vi "Handle.vi"(8 "error in (no error)":errorcluster, 11 "Instrument in":refnum<class "Instrument.lvclass">) -> (0 "error out":errorcluster, 3 "Instrument out":refnum<class "Instrument.lvclass">)   [LabVIEW 2018, in "Instrument.lvclass"]
uses:
  Instrument.lvclass
  Instrument.lvclass/Instrument.ctl
  Server/Server.lvclass
  Comm/Stream/Stream.lvclass
  Device/Optics/Opt_Selector/Opt_Selector.lvclass
  Device/Optics/Opt_Continuous/Opt_Continuous.lvclass
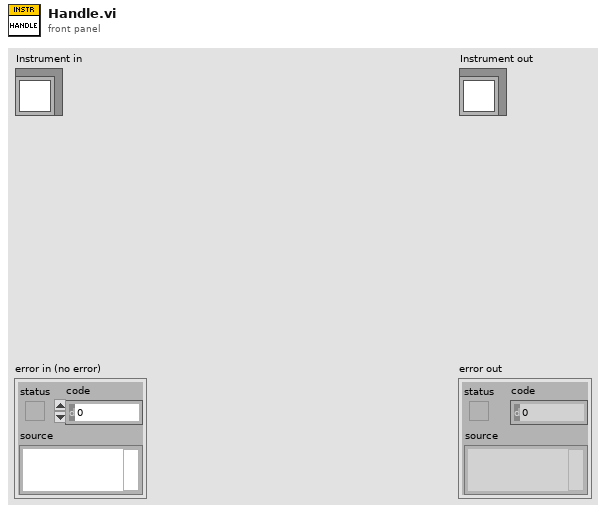
[diagram p1: front panel]
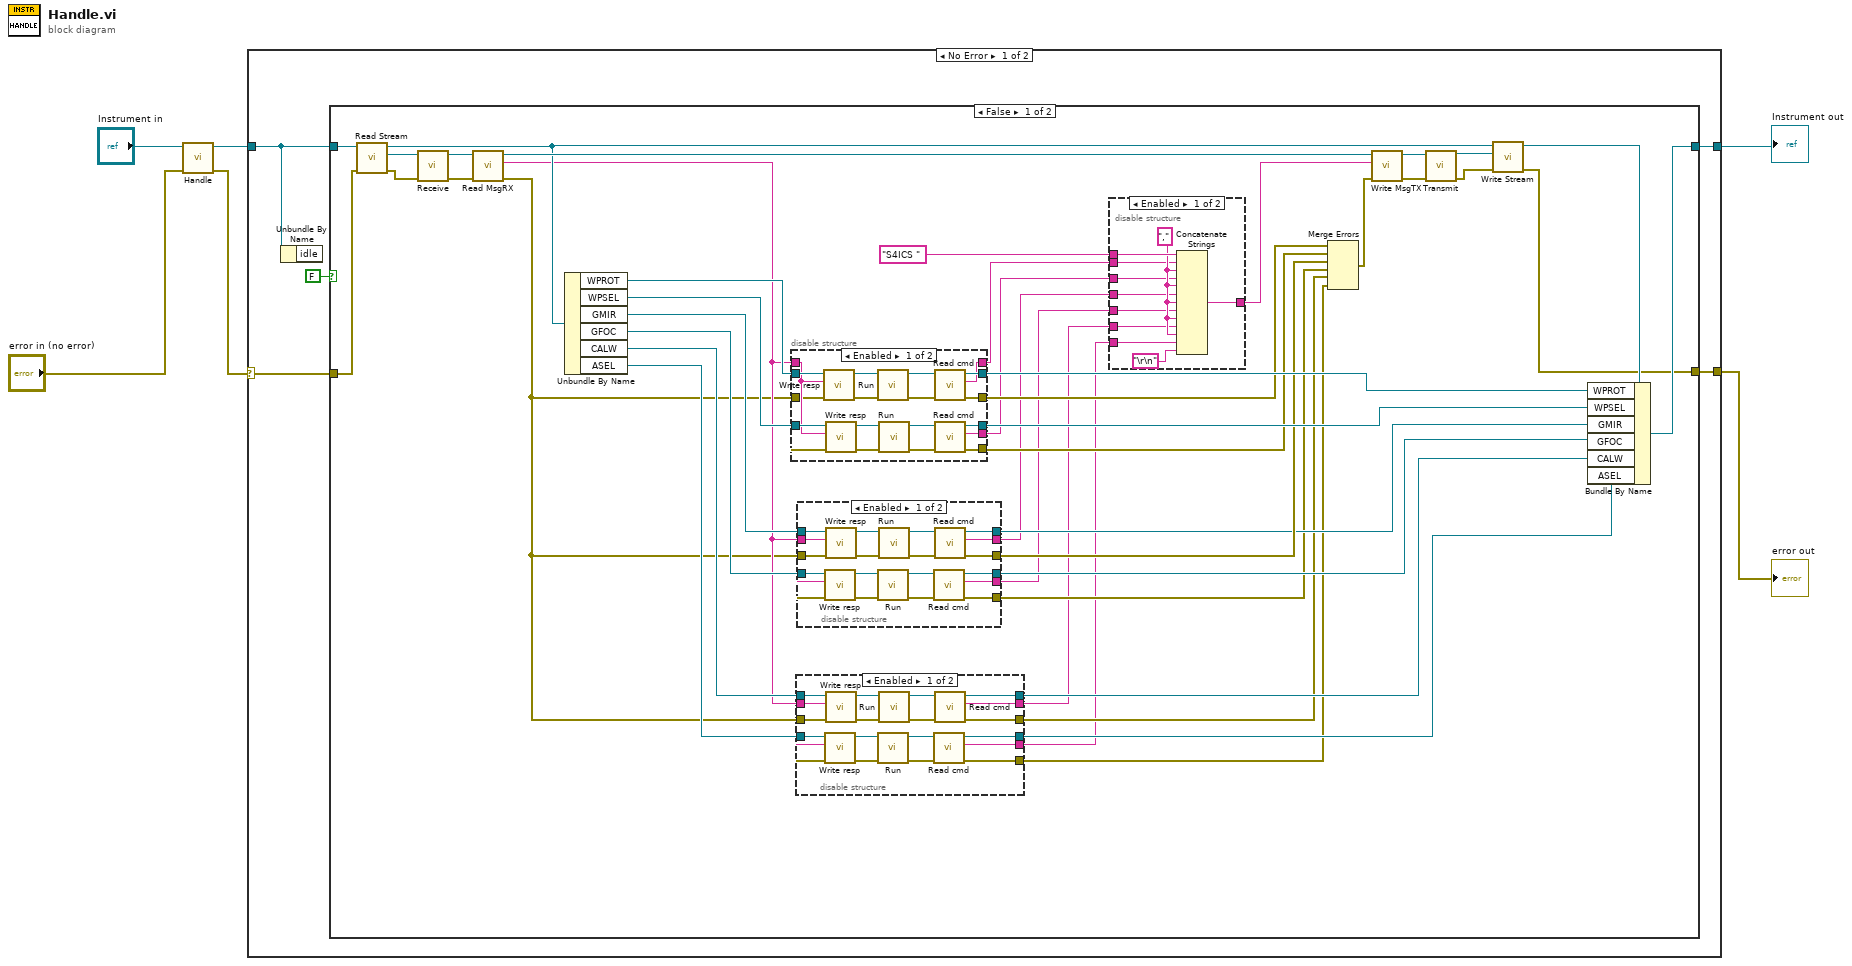
[diagram p0: block diagram]
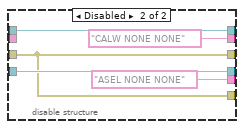
[diagram p2: hidden frame]
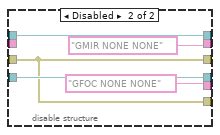
[diagram p3: hidden frame]
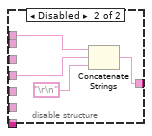
[diagram p4: hidden frame]
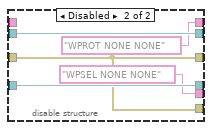
[diagram p5: hidden frame]
diagram:
  n1 = call-parent "Handle.vi"("error in (no error)"="error in (no error)", "Server in"="Instrument in") -> ("error out"=w3:errorcluster, "Server out"=w4:refnum<class "Instrument.lvclass">)  [unwired: 8 in]
  n2 = case shown="No Error" w3 {
    selector: w3 -> [w11 w142]
    tunnel: [w9 w142] -> w2
    tunnel: [w10 w141] -> w1
    tunnel: w4 -> [w8 w141]
    frame No Error {
      n3 = Unbundle By Name(w8) -> ()  [unwired: 1 out]
      n4 = case shown="False" FALSE {
        tunnel: w11 -> [w53 w139]
        tunnel: [w51 w140] -> w10
        tunnel: [w41 w139] -> w9
        tunnel: w8 -> [w19 w140]
        frame False {
          n5 = call-dynamic "Read Stream.vi"("error in (no error)"=w53, "Server in"=w19) -> ("error out"=w54:errorcluster, "Stream.lvclass"=w55:refnum<class "Stream.lvclass">, "Server out"=w45:refnum<class "Instrument.lvclass">)  [unwired: 7 in]
          n6 = call-dynamic "Receive.vi"("error in (no error)"=w54, "Stream in"=w55) -> ("error out"=w50:errorcluster, "Stream out"=w49:refnum<class "Stream.lvclass">)  [unwired: 8 in]
          n7 = call-dynamic "Read MsgRX.vi"("error in (no error)"=w50, "Comm in"=w49) -> ("error out"=w26:errorcluster, "MsgRX"=w27:string, "Comm out"=w48:refnum<class "Stream.lvclass">)  [unwired: 7 in]
          n8 = Unbundle By Name(w45) -> ("WPROT"=w52:refnum<class "Opt_Selector.lvclass">, "WPSEL"=w40:refnum<class "Opt_Selector.lvclass">, "GMIR"=w33:refnum<class "Opt_Continuous.lvclass">, "GFOC"=w30:refnum<class "Opt_Continuous.lvclass">, "CALW"=w29:refnum<class "Opt_Selector.lvclass">, "ASEL"=w28:refnum<class "Opt_Selector.lvclass">)
          n9 = disable-structure shown="Enabled" {
            disable-tunnel: w52 -> [w133 w138]
            disable-tunnel: w40 -> [w128 w137]
            disable-tunnel: [w127 w138] -> w37
            disable-tunnel: [w126 w136] -> w36
            disable-tunnel: [w125 w137] -> w35
            disable-tunnel: [w124 w136] -> w34
            disable-tunnel: w27 -> [w123 _]
            disable-tunnel: w26 -> [w122 w136]
            disable-tunnel: [w121 "WPROT NONE NONE" ("cmd")] -> w18
            disable-tunnel: [w120 "WPSEL NONE NONE" ("cmd")] -> w17
            frame Enabled {
              n10 = call-dynamic "Write resp.vi"("error in (no error)"=w122, "resp"=w123, "Device in"=w133) -> ("error out"=w131:errorcluster, "Device out"=w132:refnum<class "Opt_Selector.lvclass">)  [unwired: 7 in]
              n11 = call-dynamic "Write resp.vi"("error in (no error)"=w122, "resp"=w123, "Device in"=w128) -> ("error out"=w118:errorcluster, "Device out"=w119:refnum<class "Opt_Selector.lvclass">)  [unwired: 7 in]
              n12 = call-dynamic "Run.vi"("error in (no error)"=w131, "Opctics in"=w132) -> ("error out"=w130:errorcluster, "Opt_Selector out"=w129:refnum<class "Opt_Selector.lvclass">)  [unwired: 8 in]
              n13 = call-dynamic "Run.vi"("error in (no error)"=w118, "Opctics in"=w119) -> ("error out"=w117:errorcluster, "Opt_Selector out"=w116:refnum<class "Opt_Selector.lvclass">)  [unwired: 8 in]
              n14 = call-dynamic "Read cmd.vi"("error in (no error)"=w130, "Device in"=w129) -> ("error out"=w126:errorcluster, "cmd"=w121:string, "Device out"=w127:refnum<class "Opt_Selector.lvclass">)  [unwired: 7 in]
              n15 = call-dynamic "Read cmd.vi"("error in (no error)"=w117, "Device in"=w116) -> ("error out"=w124:errorcluster, "cmd"=w120:string, "Device out"=w125:refnum<class "Opt_Selector.lvclass">)  [unwired: 7 in]
            }
            frame Disabled {
            }
          }
          n16 = disable-structure shown="Enabled" {
            disable-tunnel: w29 -> [w73 w78]
            disable-tunnel: w28 -> [w72 w76]
            disable-tunnel: w27 -> [w71 _]
            disable-tunnel: w26 -> [w70 w74]
            disable-tunnel: [w69 w78] -> w24
            disable-tunnel: [w68 w76] -> w23
            disable-tunnel: [w67 w74] -> w21
            disable-tunnel: [w66 w74] -> w20
            disable-tunnel: [w65 "CALW NONE NONE" ("cmd")] -> w14
            disable-tunnel: [w64 "ASEL NONE NONE" ("cmd")] -> w13
            frame Enabled {
              n17 = call-dynamic "Write resp.vi"("error in (no error)"=w70, "resp"=w71, "Device in"=w72) -> ("error out"=w58:errorcluster, "Device out"=w59:refnum<class "Opt_Selector.lvclass">)  [unwired: 7 in]
              n18 = call-dynamic "Write resp.vi"("error in (no error)"=w70, "resp"=w71, "Device in"=w73) -> ("error out"=w62:errorcluster, "Device out"=w63:refnum<class "Opt_Selector.lvclass">)  [unwired: 7 in]
              n19 = call-dynamic "Run.vi"("error in (no error)"=w58, "Opctics in"=w59) -> ("error out"=w57:errorcluster, "Opt_Selector out"=w56:refnum<class "Opt_Selector.lvclass">)  [unwired: 8 in]
              n20 = call-dynamic "Run.vi"("error in (no error)"=w62, "Opctics in"=w63) -> ("error out"=w61:errorcluster, "Opt_Selector out"=w60:refnum<class "Opt_Selector.lvclass">)  [unwired: 8 in]
              n21 = call-dynamic "Read cmd.vi"("error in (no error)"=w57, "Device in"=w56) -> ("error out"=w66:errorcluster, "cmd"=w64:string, "Device out"=w68:refnum<class "Opt_Selector.lvclass">)  [unwired: 7 in]
              n22 = call-dynamic "Read cmd.vi"("error in (no error)"=w61, "Device in"=w60) -> ("error out"=w67:errorcluster, "cmd"=w65:string, "Device out"=w69:refnum<class "Opt_Selector.lvclass">)  [unwired: 7 in]
            }
            frame Disabled {
            }
          }
          n23 = disable-structure shown="Enabled" {
            disable-tunnel: w33 -> [w96 w99]
            disable-tunnel: [w95 w97] -> w32
            disable-tunnel: [w94 w99] -> w31
            disable-tunnel: w30 -> [w93 w98]
            disable-tunnel: w27 -> [w92 _]
            disable-tunnel: w26 -> [w91 w97]
            disable-tunnel: [w90 w98] -> w25
            disable-tunnel: [w89 w97] -> w22
            disable-tunnel: [w88 "GMIR NONE NONE" ("cmd")] -> w16
            disable-tunnel: [w87 "GFOC NONE NONE" ("cmd")] -> w15
            frame Enabled {
              n24 = call-dynamic "Write resp.vi"("error in (no error)"=w91, "resp"=w92, "Device in"=w93) -> ("error out"=w81:errorcluster, "Device out"=w82:refnum<class "Opt_Continuous.lvclass">)  [unwired: 7 in]
              n25 = call-dynamic "Write resp.vi"("error in (no error)"=w91, "resp"=w92, "Device in"=w96) -> ("error out"=w85:errorcluster, "Device out"=w86:refnum<class "Opt_Continuous.lvclass">)  [unwired: 7 in]
              n26 = call-dynamic "Run.vi"("error in (no error)"=w81, "Opctics in"=w82) -> ("error out"=w80:errorcluster, "Opt_Continuous out"=w79:refnum<class "Opt_Continuous.lvclass">)  [unwired: 8 in]
              n27 = call-dynamic "Run.vi"("error in (no error)"=w85, "Opctics in"=w86) -> ("error out"=w84:errorcluster, "Opt_Continuous out"=w83:refnum<class "Opt_Continuous.lvclass">)  [unwired: 8 in]
              n28 = call-dynamic "Read cmd.vi"("error in (no error)"=w80, "Device in"=w79) -> ("error out"=w89:errorcluster, "cmd"=w87:string, "Device out"=w90:refnum<class "Opt_Continuous.lvclass">)  [unwired: 7 in]
              n29 = call-dynamic "Read cmd.vi"("error in (no error)"=w84, "Device in"=w83) -> ("error out"=w95:errorcluster, "cmd"=w88:string, "Device out"=w94:refnum<class "Opt_Continuous.lvclass">)  [unwired: 7 in]
            }
            frame Disabled {
            }
          }
          n30 = disable-structure shown="Enabled" {
            disable-tunnel: "S4ICS " ("string") -> [w111 w115]
            disable-tunnel: w18 -> [w108 _]
            disable-tunnel: w17 -> [w107 _]
            disable-tunnel: w16 -> [w106 w114]
            disable-tunnel: w15 -> [w105 _]
            disable-tunnel: w14 -> [w104 _]
            disable-tunnel: w13 -> [w103 _]
            disable-tunnel: [w102 w112] -> w12
            frame Enabled {
              w110 = "," ("string")
              n31 = Concatenate Strings(w111, w108, w110, w107, w110, w106, w110, w105, w110, w104, w110, w103, "\r\n") -> (w102:string)
            }
            frame Disabled {
              n32 = Concatenate Strings(w115, w114, "\r\n") -> (w112:string)
            }
          }
          n33 = Merge Errors(w36, w34, w32, w22, w21, w20) -> (w39:errorcluster)
          n34 = call-dynamic "Write MsgTX.vi"("error in (no error)"=w39, "MsgTX"=w12, "Comm in"=w48) -> ("error out"=w46:errorcluster, "Comm out"=w47:refnum<class "Stream.lvclass">)  [unwired: 7 in]
          n35 = call-dynamic "Transmit.vi"("error in (no error)"=w46, "Stream in"=w47) -> ("error out"=w42:errorcluster, "Stream out"=w44:refnum<class "Stream.lvclass">)  [unwired: 8 in]
          n36 = call-dynamic "Write Stream.vi"("error in (no error)"=w42, "Stream.lvclass"=w44, "Server in"=w45) -> ("error out"=w41:errorcluster, "Server out"=w43:refnum<class "Instrument.lvclass">)  [unwired: 7 in]
          n37 = Bundle By Name(cluster=w43, "WPROT"=w37, "WPSEL"=w35, "GMIR"=w31, "GFOC"=w25, "CALW"=w24, "ASEL"=w23) -> (w51:refnum<class "Instrument.lvclass">)
        }
        frame True {
        }
      }
    }
    frame Error {
    }
  }
  "error out" <- w2
  "Instrument out" <- w1
